vi "Read_semaphore.vi"(8 "error in (no error)":errorcluster, 11 "PrepLineObject in":refnum<class "PrepLineObject.lvclass">) -> (0 "error out":errorcluster, 2 "semaphore":T1, 3 "PrepLineObject out":refnum<class "PrepLineObject.lvclass">)   [LabVIEW 2018, in "PrepLineObject.lvclass"]
uses:
  PrepLineObject.lvclass
  PrepLineObject.lvclass/PrepLineObject.ctl
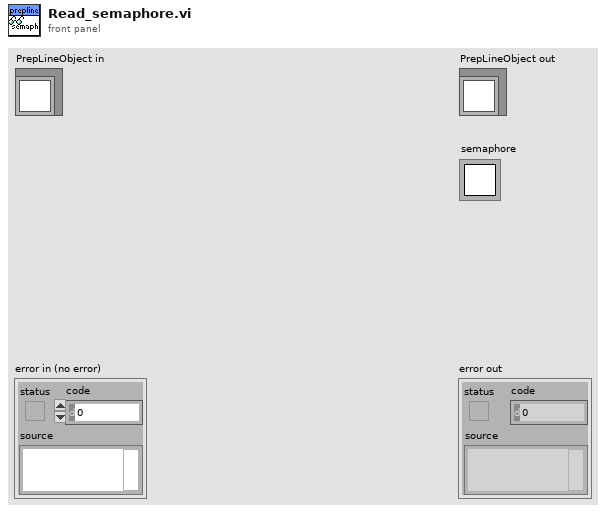
[diagram p1: front panel]
types:
  T1 = typedef "Semaphore RefNum" = refnum<k1>
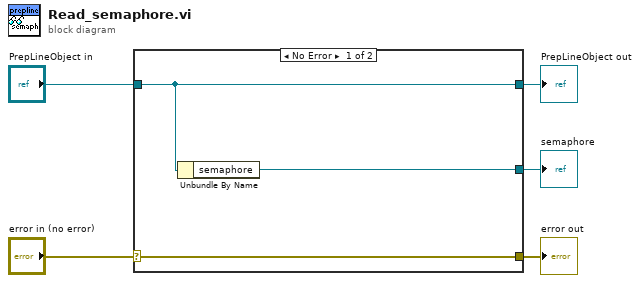
[diagram p0: block diagram]
diagram:
  n1 = case shown="No Error" "error in (no error)" {
    selector: "error in (no error)" -> [w8 w9]
    tunnel: [w8 w9] -> w4
    tunnel: [w7 w10] -> w2
    tunnel: "PrepLineObject in" -> [w7 w10]
    tunnel: [w6 _] -> w1
    frame No Error {
      n2 = Unbundle By Name(w7) -> ("semaphore"=w6:T1)
    }
    frame Error {
    }
  }
  "error out" <- w4
  "PrepLineObject out" <- w2
  "semaphore" <- w1
